vi "Get Signals Classification.vi"(8 "error in (no error)":errorcluster, 11 "Module in":refnum<class "Module.lvclass">) -> (0 "error out":errorcluster, 2 "Classifications":string[](array[string]), 3 "Module out":refnum<class "Module.lvclass">)   [LabVIEW 2025, in "Module.lvclass"]
doc: "Get all signal types that are being used."
uses:
  Module.lvclass
  Module.lvclass/Module.ctl
  Signal/Signal/Signal.lvclass
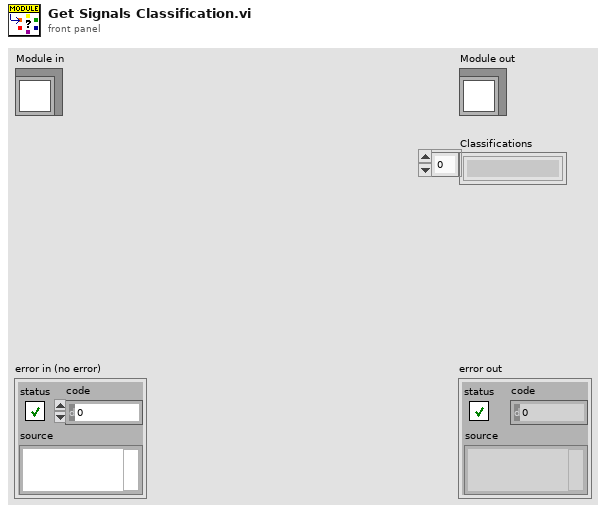
[diagram p1: front panel]
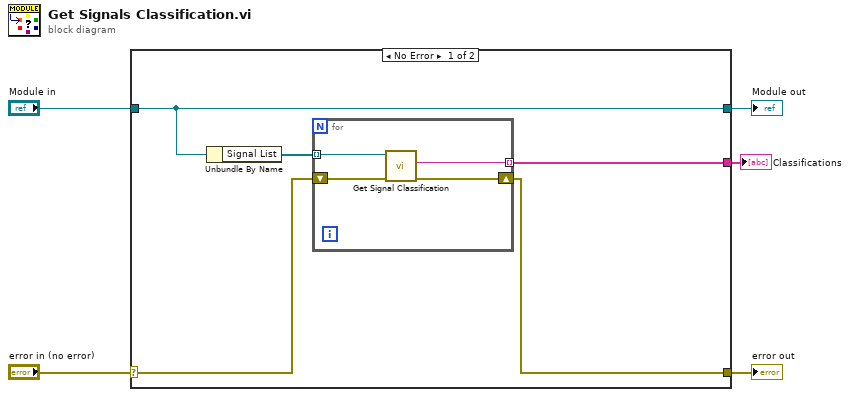
[diagram p0: block diagram]
diagram:
  n1 = case shown="No Error" "error in (no error)" {
    selector: "error in (no error)" -> [w8 w16]
    tunnel: [w7 w16] -> w4
    tunnel: [w9 w15] -> w2
    tunnel: "Module in" -> [w9 w15]
    tunnel: [w6 _] -> w1
    frame No Error {
      n2 = Unbundle By Name(w9) -> ("Signal List"=w10:refnum<class "Signal.lvclass">[])
      n3 = for {
        tunnel: w10 -> [w13] mode=indexing
        tunnel: [w11] -> w6 mode=indexing
        shift-right: [w12] -> w7
        shift-left: w8 -> [w14]
        n4 = call "Get Signal Classification.vi"("error in (no error)"=w14, "IO Class in"=w13) -> ("error out"=w12:errorcluster, "Classification"=w11:string)  [unwired: 7 in, 1 out]
      }
    }
    frame Error {
    }
  }
  "error out" <- w4
  "Module out" <- w2
  "Classifications" <- w1
